vi "moterVelControl.vi"(7 "Motor ID":T1, 8 "error in":errorcluster, 9 "reset?":bool, 10 "Speed (deg/s)":dbl, 11 "TitanQuad Object":refnum<class "TitanQuad.lvclass">) -> (0 "error out":errorcluster, 3 "TitanQuad Object 2":refnum<class "TitanQuad.lvclass">)   [LabVIEW 2020]
uses:
  <vilib>/CISH Robotics/L4VMX TitanQuad/TitanQuad.lvclass
  <vilib>/CISH Robotics/L4VMX TitanQuad/Motor ID.ctl
  <vilib>/addons/control/pid/pid.llb/PID (DBL).vi
  <vilib>/addons/control/pid/NI_PID_pid.lvlib
panel:
  out "output":dbl format="%.2f"
  in  "dt":dbl=50.0 format="%#_13g"
  in  "PID gains":T2={"proportional gain (Kc)"=1.6, "integral time (Ti, min)"=0.0, "derivative time (Td, min)"=0.0003}
  out "ENC (deg)":dbl
  out "waveForm":cluster{"targetPos":dbl, "ENC (deg)":dbl}
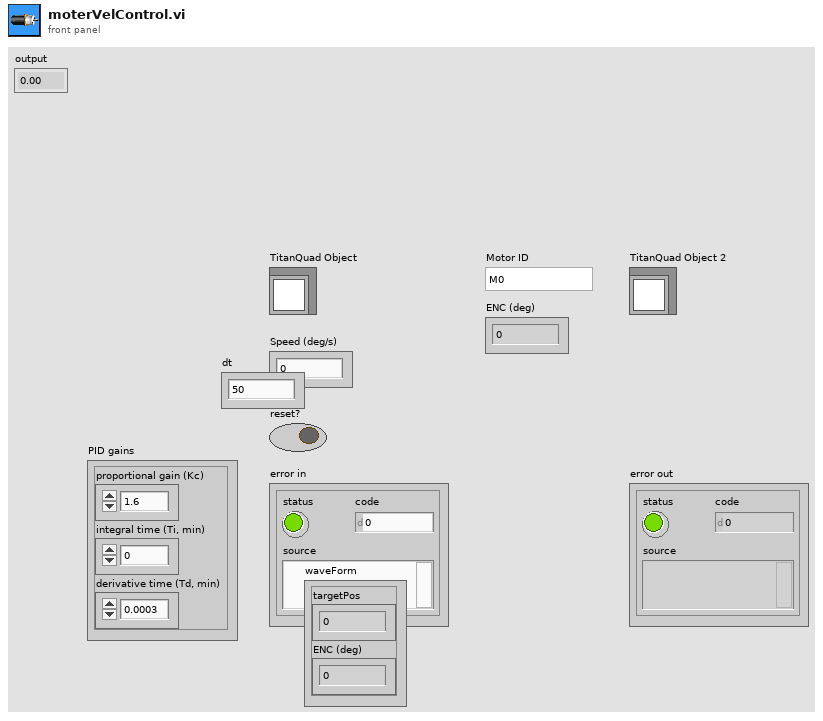
[diagram p1: front panel]
types:
  T1 = typedef "TitanQuad.lvlib/TitanQuad.lvclass/Motor ID.ctl" = enum16{"M0", "M1", "M2", "M3"}
  T2 = cluster{"proportional gain (Kc)":dbl, "integral time (Ti, min)":dbl, "derivative time (Td, min)":dbl}
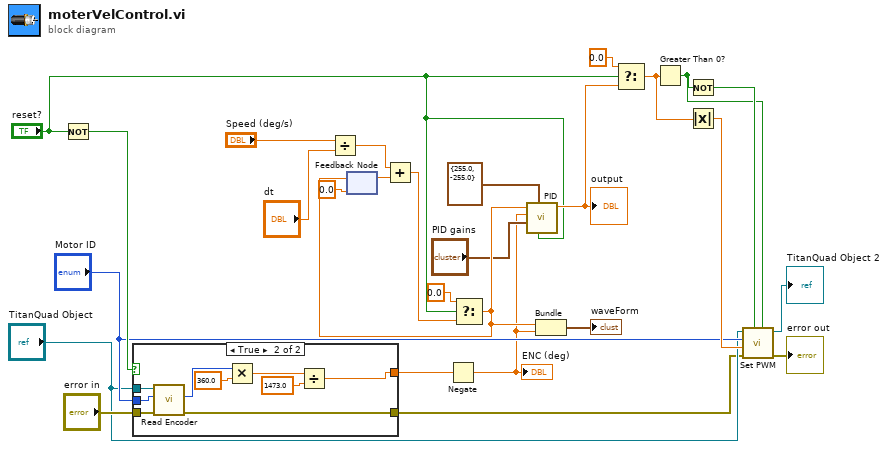
[diagram p0: block diagram]
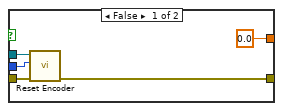
[diagram p2: hidden frame]
diagram:
  n1 = Not(x="reset?") -> (.not. x?=w11:bool)
  n2 = case shown="True" w11 {
    tunnel: "error in" -> [w29 w37]
    tunnel: [w30 w36] -> w2
    tunnel: [0.0 w35] -> w13
    tunnel: "Motor ID" -> [w32 w34]
    tunnel: "TitanQuad Object" -> [w31 w33]
    frame False {
      n3 = call <vilib>:"Reset Encoder.vi"("Error In"=w29, "Motor ID"=w32, "TitanQuad Object"=w31) -> ("Error Out"=w30:errorcluster)  [unwired: 7 in, 1 out]
    }
    frame True {
      n4 = call <vilib>:"Read Encoder.vi"("Error In"=w37, "Motor ID"=w34, "TitanQuad Object"=w33) -> ("Error Out"=w36:errorcluster, "Counter Value"=w38:i32)  [unwired: 6 in, 1 out]
      n5 = Multiply(x=w38, y=360.0) -> (x*y=w39:dbl)
      n6 = Divide(x=w39, y=1473.0) -> (x/y=w35:dbl)
    }
  }
  n7 = Divide(x="Speed (deg/s)", y="dt") -> (x/y=w21:dbl)
  n8 = feedback #1(0.0 ("t")) -> (w22:dbl)
  n9 = Add(x=w21, y=w22) -> (x+y=w26:dbl)
  n10 = Negate(x=w13) -> (-x=w1:dbl)
  "ENC (deg)" <- w1
  n11 = Select(t=0.0, s="reset?", f=w26) -> (s? t:f=w27:dbl)
  n12 = feedback-in #1(w27) -> ()
  n13 = call-poly <vilib>:"PID.vi"("reinitialize? (F)"="reset?", "output range"=cluster{"output high":dbl, "output low":dbl} {"output high"=255.0, "output low"=-255.0}, "PID gains"="PID gains", "process variable"=w1, "setpoint"=w27) -> ("output"=w24:dbl)  [unwired: 5 in, 1 out]
  "output" <- w24
  n14 = Bundle("t"=w27, w1) -> (→"waveForm":cluster{"t":dbl, dbl})  [unwired: 1 in]
  n15 = Select(t=0.0, s="reset?", f=w24) -> (s? t:f=w7:dbl)
  n16 = Greater Than 0?(x=w7) -> (x > 0?=w8:bool)
  n17 = Not(x=w8) -> (.not. x?=w9:bool)
  n18 = Absolute Value(x=w7) -> (abs(x)=w10:dbl)
  n19 = call <vilib>:"Set PWM.vi"("Dir B"=w8, "Dir A"=w9, "Error In"=w2, "Duty Cycle (0~255)"=w10, "Motor ID"="Motor ID", "TitanQuad Object"="TitanQuad Object") -> ("Error Out"=→"error out":errorcluster, "TitanQuad Object"=→"TitanQuad Object 2":refnum<class "TitanQuad.lvclass">)  [unwired: 4 in]
